vi "Initialize.vi"(8 "error in (no error)":errorcluster, 11 "Camera_Prime95B in":refnum<class "Camera_Prime95B.lvclass">) -> (0 "error out":errorcluster, 3 "Camera_Prime95B out":refnum<class "Camera_Prime95B.lvclass">)   [LabVIEW 2020, in "Camera_Prime95B.lvlib" / "Camera_Prime95B.lvclass"]
uses:
  Camera_Prime95B.lvclass
  E:/Development/DevHardSoftware/MMicroscopyAF/Model/Real Hardware/Camera_Prime95B/Camera_Prime95B/Dependencies/PVCamNET.dll
  Dependencies/PVCamNET.dll
  Camera_Prime95B.lvclass/Camera_Prime95B.ctl
  HAL Layer/Component/Camera/Camera/Camera.lvclass
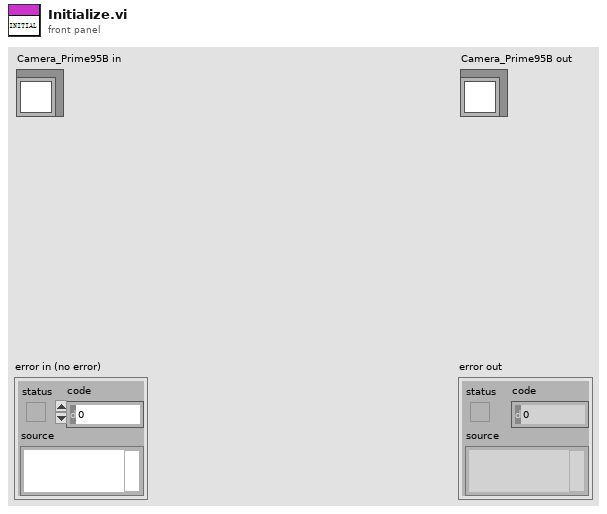
[diagram p1: front panel]
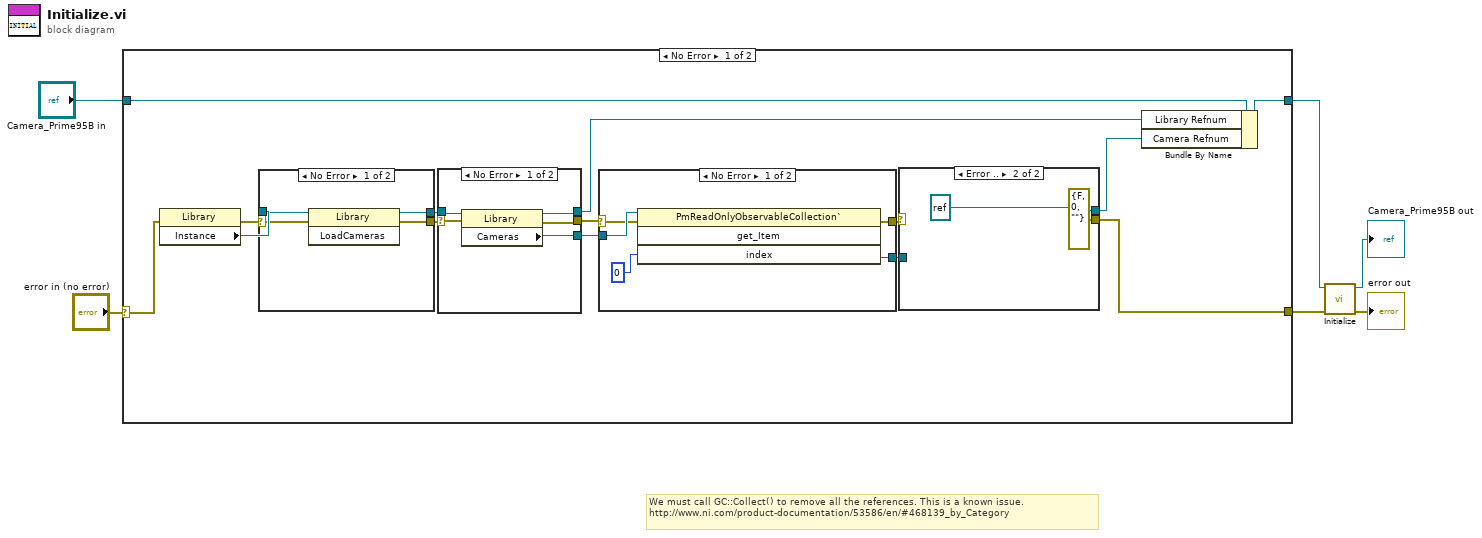
[diagram p0: block diagram]
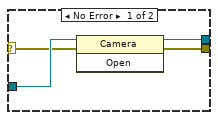
[diagram p2: hidden frame]
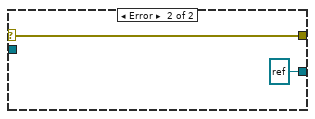
[diagram p3: hidden frame]
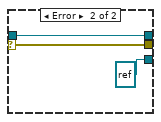
[diagram p4: hidden frame]
diagram:
  # "We must call GC::Collect() to remove all the references. This is a known issue.\nhttp://www.ni.com/product-documentation/53586/en/#468139_by_Category"
  n1 = case shown="No Error" "error in (no error)" {
    selector: "error in (no error)" -> [w12 w49]
    tunnel: [w11 w49] -> w3
    tunnel: "Camera_Prime95B in" -> [w10 w48]
    tunnel: [w9 w48] -> w1
    frame No Error {
      n2 = property class="Library"(error in=w12) -> (error out=w20:errorcluster, "Instance"=w17:refnum<k24>)  [unwired: 1 in, 1 out]
      n3 = case shown="No Error" w20 {
        selector: w20 -> [w43 w47]
        tunnel: [w44 w47] -> w18
        tunnel: [w45 w46] -> w19
        tunnel: w17 -> [w42 w46]
        frame No Error {
          n4 = invoke class="Library" method="LoadCameras"(reference=w42, error in=w43) -> (reference out=w45:refnum<k24>, error out=w44:errorcluster)  [unwired: 1 in, 1 out]
        }
        frame Error {
        }
      }
      n5 = case shown="No Error" w18 {
        selector: w18 -> [w38 w41]
        tunnel: [w35 w41] -> w14
        tunnel: w19 -> [w37 w40]
        tunnel: [w36 w40] -> w8
        tunnel: [w34 refnum<k24> refnum ("Cameras")] -> w16
        frame No Error {
          n6 = property class="Library"(reference=w37, error in=w38) -> (reference out=w36:refnum<k24>, error out=w35:errorcluster, "Cameras"=w34:refnum<k24>)
        }
        frame Error {
        }
      }
      n7 = case shown="No Error" w14 {
        selector: w14 -> [w28 w33]
        tunnel: w16 -> [w31 _]
        tunnel: [w29 refnum<k24> refnum ("get_Item")] -> w15
        tunnel: [w27 w33] -> w13
        frame No Error {
          n8 = invoke class="PmReadOnlyObservableCollection`" method="get_Item"(reference=w31, error in=w28, "index"=0) -> (error out=w27:errorcluster, "get_Item"=w29:refnum<k24>)  [unwired: 1 in, 2 out]
        }
        frame Error {
        }
      }
      n9 = case shown="Error .." w13 {
        selector: w13 -> [w22 _]
        tunnel: [w21 errorcluster {"status"=FALSE, "code"=0, "source"=""} ("error out")] -> w11
        tunnel: w15 -> [w24 _]
        tunnel: [w23 refnum<k24> refnum ("get_Item")] -> w7
        frame No Error {
          n10 = invoke class="Camera" method="Open"(reference=w24, error in=w22) -> (reference out=w23:refnum<k24>, error out=w21:errorcluster)  [unwired: 1 in, 1 out]
        }
        frame Error {
        }
      }
      n11 = Bundle By Name(cluster=w10, "Library Refnum"=w8, "Camera Refnum"=w7) -> (w9:refnum<class "Camera_Prime95B.lvclass">)
    }
    frame Error {
    }
  }
  n12 = call-parent "Initialize.vi"("error in (no error)"=w3, "Device in"=w1) -> ("error out"=→"error out":errorcluster, "Device out"=→"Camera_Prime95B out":refnum<class "Camera_Prime95B.lvclass">)  [unwired: 8 in]
